vi "PH_Beckhoff_PP_PU.set HV Meas GUI Elements to Default.vi"(0 "i ref in":refnum<vi>, 2 "PUs":T1[](array[typedef]), 5 "error in":errorcluster) -> (14 "i ref out":refnum<vi>, 19 "error out":errorcluster)   [LabVIEW 2014, in "PH_Beckhoff_PP_PU.lvlib"]
uses:
  PH_Beckhoff_PP_PU.lvlib
  PH_Basics/PH_PP_Common/PH_PP_Common.PUs.ctl
  PH_Beckhoff_PP_PU.HV Meas Tags.ctl
  PH_Basics/PH_Common/PH_Common.lvlib
  PH_Basics/PH_PP_Common/PH_PP_Common.lvlib
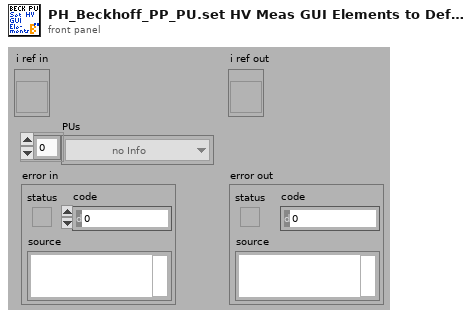
[diagram p1: front panel]
types:
  T1 = typedef "PH_PP_Common.lvlib/PH_PP_Common.PUs.ctl" = enum16{"no Info", "PA-19mm-1", "PA-19mm-2", "PA-45mm-PILC", "PA-45mm-MAIN", "MA-PU-1", "MA-PU-2", "MA-PU-3", "MA-PU-4", "MA-PU-5", "MA-PU-6", "MA-FR", "MA-PILC", "PA-45mm-DP"}
  T2 = typedef "PH_Beckhoff_PP_PU.lvlib/PH_Beckhoff_PP_PU.i attribute.ctl" = cluster{"HV Meas":cluster{"Input GUI Ref":refnum<vi>, "Voltage Service ID":i32, "Voltage [V]":dbl, "Quality":bool, "# in Data":i32}[], "Trigger":cluster{"Status":cluster{"GUI Ref":refnum<vi>, "Status Service ID":i32, "Status":T3}, "last shot:":cluster{"GUI Ref":refnum<vi>, "Service ID":i32, "Time":string}, "DIs":cluster{"triggered":cluster{"GUI Ref":refnum<vi>, "# in Data":i32}, "fired":cluster{"GUI Ref":refnum<vi>, "# in Data":i32}}, "GUI Ref Indicator":refnum<vi>}[], "RR":cluster{"Status":cluster{"GUI Ref":refnum<vi>, "Status Service ID":i32, "Status":T3}, "DIs":cluster{"closed":cluster{"GUI Ref":refnum<vi>, "# in Data":i32}, "open":cluster{"GUI Ref":refnum<vi>, "# in Data":i32}}, "Close":cluster{"GUI Ref":refnum<vi>, "# in Data":i32}, "GUI Ref Indicator":refnum<vi>}[], "Igni":cluster{"Status":cluster{"GUI Ref":refnum<vi>, "Status Service ID":i32, "Status":T3}, "DIs":cluster{"heating on":cluster{"GUI Ref":refnum<vi>, "# in Data":i32}, "water on":cluster{"GUI Ref":refnum<vi>, "# in Data":i32}}, "Device on":cluster{"GUI Ref":refnum<vi>, "# in Data":i32}, "GUI Ref Indicator":refnum<vi>}[], "PSU":cluster{"Status":cluster{"GUI Ref":refnum<vi>, "Status Service ID":i32, "Status":T3}, "Limit Service ID":i32, "DIs":cluster{"inhibit":cluster{"GUI Ref":refnum<vi>, "# in Data":i32}, "end of charge":cluster{"GUI Ref":refnum<vi>, "# in Data":i32}, "HV on":cluster{"GUI Ref":refnum<vi>, "# in Data":i32}, "overtemp":cluster{"GUI Ref":refnum<vi>, "# in Data":i32}, "interlock":cluster{"GUI Ref":refnum<vi>, "# in Data":i32}, "load fault":cluster{"GUI Ref":refnum<vi>, "# in Data":i32}, "sum fault":cluster{"GUI Ref":refnum<vi>, "# in Data":i32}, "HV off":cluster{"GUI Ref":refnum<vi>, "# in Data":i32}, "DC ok":cluster{"GUI Ref":refnum<vi>, "# in Data":i32}}, "AIs":cluster{"voltage":cluster{"GUI Ref":refnum<vi>, "# in Data":i32}, "current":cluster{"GUI Ref":refnum<vi>, "# in Data":i32}}, "DAs":cluster{"inhibit":cluster{"GUI Ref":refnum<vi>, "# in Data":i32}, "interlock":cluster{"GUI Ref":refnum<vi>, "# in Data":i32}, "HV on":cluster{"GUI Ref":refnum<vi>, "# in Data":i32}, "Reset":cluster{"GUI Ref":refnum<vi>, "# in Data":i32}}, "AAs":cluster{"Voltage to set":cluster{"GUI Ref":refnum<vi>, "# in Data":i32}}, "GUI Ref Indicator":refnum<vi>}[], "reconfigured":cluster{"?":bool, "GUI Ref":refnum<vi>}, "PU Rack Type":T4, "HV Meas Info":T5, "PSU Info":T6}
  T3 = typedef "PH_StatusHandler.lvlib/PH_StatusHandler.Status.ctl" = i16
  T4 = typedef "PH_Beckhoff_PP_PU.lvlib/PH_Beckhoff_PP_PU.PU Rack Type.ctl" = enum16{"no Info", "PA 19mm", "PA 45mm", "MA PU 1 and 2", "MA PU 3 and 4", "MA PU 5 and 6", "MA FR and PILC"}
  T5 = typedef "PH_Beckhoff_PP_PU.lvlib/PH_Beckhoff_PP_PU.HV Meas Info.ctl" = cluster{"Period Time [s]":dbl, "Subtractor 1 [Hz]":dbl, "Devider 1 [Hz/kV]":dbl, "Subtractor 2 [Hz]":dbl, "Devider 2 [Hz/kV]":dbl}
  T6 = typedef "PH_Beckhoff_PP_PU.lvlib/PH_Beckhoff_PP_PU.PSU Info.ctl" = cluster{"Limits 1 [V]":cluster{"Lower":dbl, "Upper":dbl}, "Limits 2 [V]":cluster{"Lower":dbl, "Upper":dbl}}
  T7 = cluster{"Input GUI Ref":refnum<vi>, "Voltage Service ID":i32, "Voltage [V]":dbl, "Quality":bool, "# in Data":i32}[]
  T8 = typedef "PH_Beckhoff_PP_PU.lvlib/PH_Beckhoff_PP_PU.HV Meas Tags.ctl" = enum16{"voltage-raw", "voltage"}
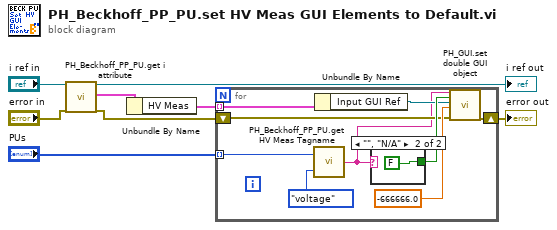
[diagram p0: block diagram]
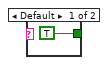
[diagram p2: hidden frame]
diagram:
  n1 = call "PH_Beckhoff_PP_PU.get i attribute.vi"("i ref in"="i ref in", "error in (no error)"="error in") -> ("i ref out"=→"i ref out":refnum<vi>, "i attribute"=w6:T2, "error out"=w4:errorcluster)  [unwired: 15 in]
  n2 = Unbundle By Name(w6) -> ("HV Meas"=w5:T7)
  n3 = for {
    tunnel: w5 -> [w16] mode=indexing
    shift-right: [w17] -> w7
    shift-left: w4 -> [w12]
    tunnel: "PUs" -> [w10] mode=indexing
    n4 = call "PH_Beckhoff_PP_PU.get HV Meas Tagname.vi"("HV Meas Tag"=PH_Beckhoff_PP_PU.HV_Meas_Tags."voltage", "PU"=w10) -> ("HV Meas Tagname"=w9:string)
    n5 = Unbundle By Name(w16) -> ("Input GUI Ref"=w13:refnum<vi>)
    n6 = case shown="\"\", \"N/A\"" w9 {
      tunnel: [TRUE FALSE] -> w14
      frame Default {
      }
      frame "", "N/A" {
      }
    }
    n7 = call "PH_GUI.set double GUI object.vi"("Caption"=w9, "visible (true)"=w14, "GUI object Ref"=w13, "value"=-666666.0, "error in (no error)"=w12) -> ("error out"=w17:errorcluster)  [unwired: 14 in]
  }
  "error out" <- w7
